vi "tdmsGenToolAllDataTypes.vi"() -> ()   [LabVIEW 2026]
uses:
  <vilib>/platform/TimedLoop/XDataNode/XDataNode.xnode
  <vilib>/Platform/TimedLoop/XDataNode/nitl_modes.ctl
  <vilib>/Platform/TimedLoop/XDataNode/XDNodeRunTimeDep.lvlib
  <vilib>/Platform/TimedLoop/XDataNode/wakeup.ctl
  <vilib>/Platform/TimedLoop/XDataNode/timing_clust.ctl
  <vilib>/DAQmx/configure/timing.llb/DAQmx Timing (Sample Clock).vi
  <vilib>/DAQmx/configure/task.llb/DAQmx Configure Logging (TDMS).vi
  <vilib>/DAQmx/create/channels.llb/DAQmx Create Channel (AI-Voltage-Basic).vi
panel:
  in  "physical channels 2":tag
  in  "number of loops":i32=1
  in  "file format version (2.0)":enum16{"1.0", "2.0"}(ring)=enum."2.0"
  in  "create index file? (T)":bool=TRUE
  in  "byte order (2:little-endian)":T1(ring)
  in  "physical channels":tag[](array[tag])
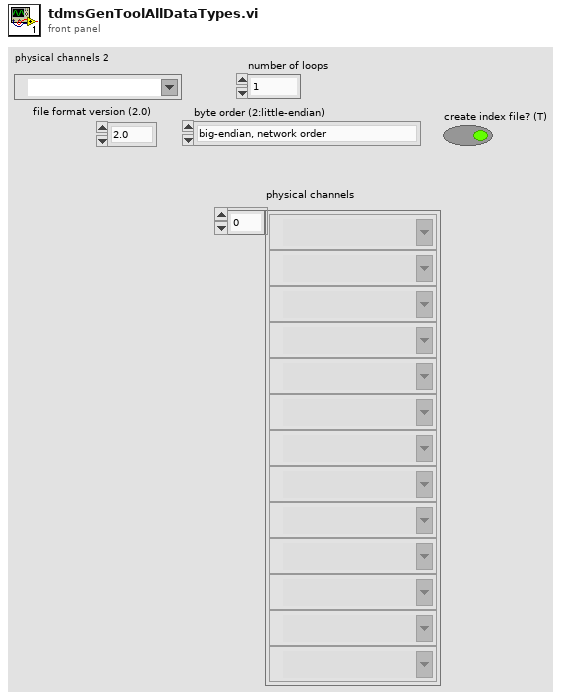
[diagram p1: front panel]
types:
  T1 = enum16{"big-endian, network order", "native, host order", "little-endian"}
  T2 = enum16{"open", "open or create", "create or replace", "create", "open (read-only)"}
  T3 = typedef "XDNodeRunTimeDep.lvlib/nitl_modes.ctl" = enum32{"No Change", "Process missed periods, maintain original phase", "Discard missed periods, maintain original phase", "Process missed periods, ignore original phase", "Discard missed periods, ignore original phase"}
  T4 = typedef "XDNodeRunTimeDep.lvlib/timing_clust.ctl" = cluster{"Expected End [f-1]":u64, "Actual End [f-1]":u64, "Finished Late? [f-1]":bool, "Expected End [i-1]":u64, "Actual End [i-1]":u64, "Finished Late? [i-1]":bool, "Expected Start [i]":u64, "Actual Start [i]":u64, "Expected Start [f]":u64, "Actual Start [f]":u64, "Source Name":string, "Structure Name":string, "Period":i64, "Deadline":i64, "Offset":i64, "Start":i64, "Priority":i32, "Timeout":i32, "Mode":T3, "Wakeup Reason":T5, "Error":errorcluster, "Source Type":string, "Secondary Source Type":string, "Global End Time":u64, "Global Start Time":u64, "Frame Duration":u64, "Iteration Duration":u64, "Assigned CPU":i32, "I/O Scan Engine Mode":u32}
  T5 = typedef "XDNodeRunTimeDep.lvlib/wakeup.ctl" = enum32{"Normal", "Aborted", "Asynchronous wakeup", "Timing source error", "Timed loop error", "Timeout"}
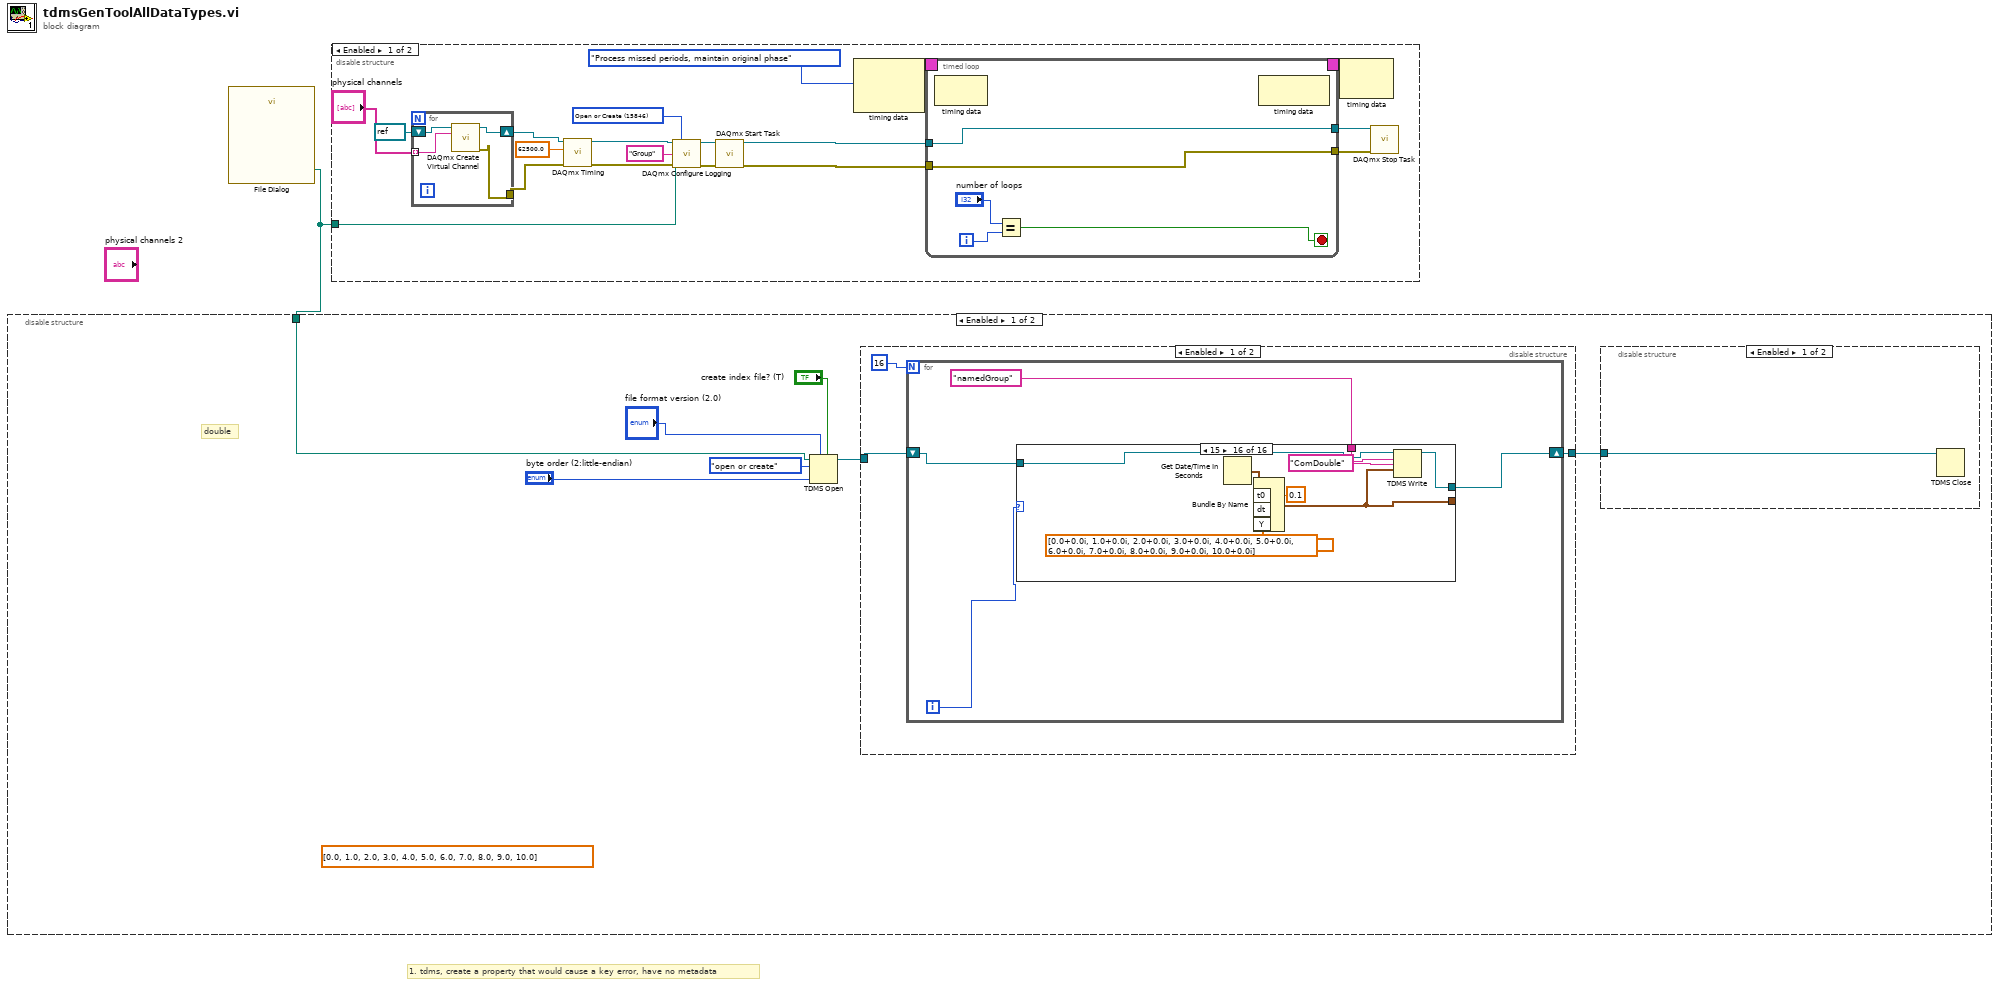
[diagram p0: block diagram]
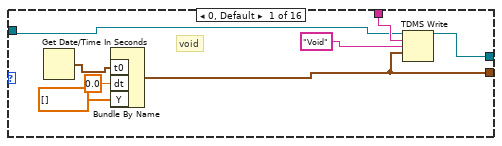
[diagram p3: hidden frame]
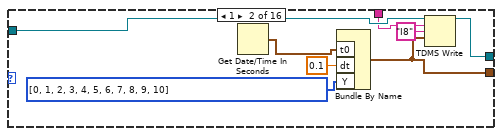
[diagram p4: hidden frame]
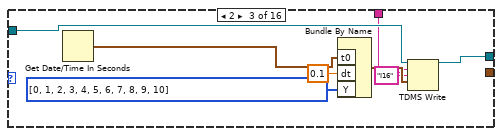
[diagram p5: hidden frame]
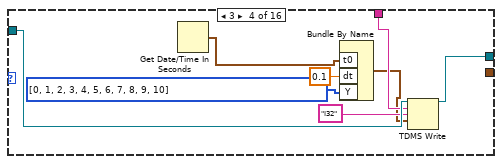
[diagram p6: hidden frame]
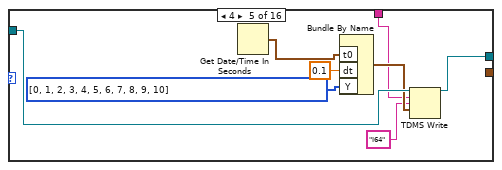
[diagram p7: hidden frame]
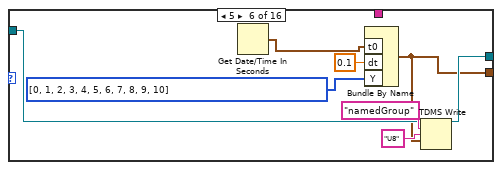
[diagram p8: hidden frame]
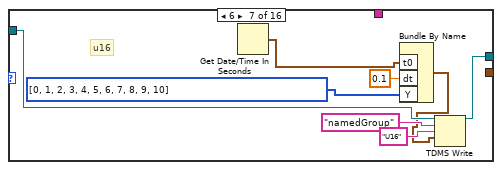
[diagram p9: hidden frame]
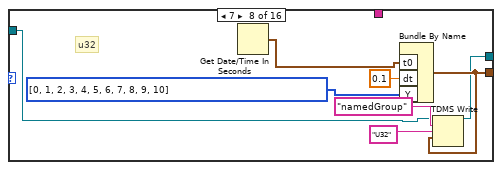
[diagram p10: hidden frame]
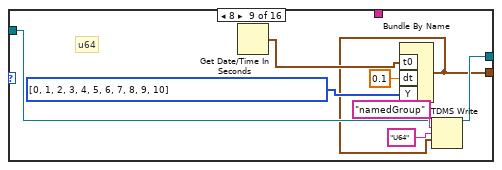
[diagram p11: hidden frame]
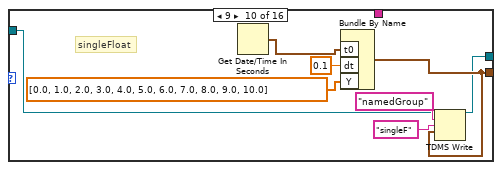
[diagram p12: hidden frame]
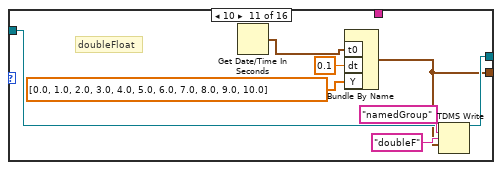
[diagram p13: hidden frame]
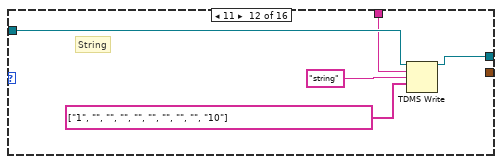
[diagram p14: hidden frame]
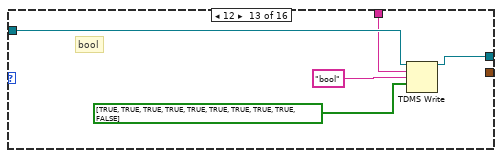
[diagram p15: hidden frame]
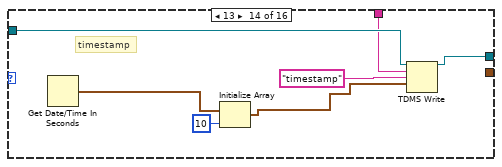
[diagram p16: hidden frame]
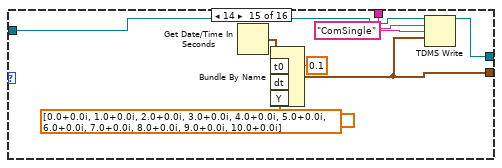
[diagram p17: hidden frame]
diagram:
  # "1. tdms, create a property that would cause a key error, have no metadata"
  n1 = call "File Dialog"() -> ("selected path"=w1:path)  [unwired: 12 in, 3 out]
  n2 = disable-structure shown="Enabled" {
    disable-tunnel: w1 -> [w6 _]
    frame Enabled {
      (unwired) sgl[] [0.0, 1.0, 2.0, 3.0, 4.0, 5.0, 6.0, 7.0, 8.0, 9.0, 10.0] ("Y")
      # "double"
      n3 = TDMS Open(5:"create index file? (T)", 7:"file format version (2.0)", 9:"byte order (2:little-endian)", 10:T2."open or create" ("operation (0:open)"), 11:w6) -> (3:w8:refnum<k34>)  [unwired: 2 in, 1 out]
      n4 = disable-structure shown="Enabled" {
        disable-tunnel: w8 -> [w11 w137]
        disable-tunnel: [w10 w137] -> w2
        frame Enabled {
          n5 = for {
            N: 16 -> [_]
            shift-right: [w14] -> w10
            shift-left: w11 -> [w15]
            i -> [w12]
            n6 = case shown="15" w12 {
              tunnel: [w19 w28 _ _ _ w56 _ w74 w80 w90 w96 _ _ _ w121 w129] -> _
              tunnel: w15 -> [w16 w26 w35 w44 w52 w58 w66 w72 w82 w88 w97 w107 w113 w120 w125 w133]
              tunnel: [w17 w27 w34 w43 w51 w57 w65 w73 w81 w89 w98 w106 w112 w119 w126 w134] -> w14
              tunnel: "namedGroup" ("group name in (Untitled)") -> [w20 w25 w33 w42 w49 _ _ _ _ _ _ w105 w111 w118 w124 w132]
              frame 0, Default {
                # "void"
                n7 = Get Date/Time In Seconds() -> (seconds since 1Jan1904=w23:timestamp)
                n8 = Bundle By Name("t0"=w23, "dt"=0.0, "Y"=dbl[] []) -> (w19:waveform(dbl))  [unwired: 1 in]
                n9 = TDMS Write(0:w16, 5:w20, 7:"Void", 9:w19) -> (4:w17:refnum<k34>)  [unwired: 2 in, 3 out]
              }
              frame 1 {
                n10 = Get Date/Time In Seconds() -> (seconds since 1Jan1904=w31:timestamp)
                n11 = Bundle By Name("t0"=w31, "dt"=0.1, "Y"=i8[] [0, 1, 2, 3, 4, 5, 6, 7, 8, 9, 10]) -> (w28:waveform(i8))  [unwired: 1 in]
                n12 = TDMS Write(0:w26, 5:w25, 7:"I8" ("channel name(s) in (Untitled)"), 9:w28) -> (4:w27:refnum<k34>)  [unwired: 2 in, 3 out]
              }
              frame 2 {
                n13 = Get Date/Time In Seconds() -> (seconds since 1Jan1904=w39:timestamp)
                n14 = Bundle By Name("t0"=w39, "dt"=0.1, "Y"=i16[] [0, 1, 2, 3, 4, 5, 6, 7, 8, 9, 10]) -> (w36:waveform(i16))  [unwired: 1 in]
                n15 = TDMS Write(0:w35, 5:w33, 7:"I16" ("channel name(s) in (Untitled)"), 9:w36) -> (4:w34:refnum<k34>)  [unwired: 2 in, 3 out]
              }
              frame 3 {
                n16 = Get Date/Time In Seconds() -> (seconds since 1Jan1904=w47:timestamp)
                n17 = Bundle By Name("t0"=w47, "dt"=0.1, "Y"=i32[] [0, 1, 2, 3, 4, 5, 6, 7, 8, 9, 10]) -> (w40:waveform(i32))  [unwired: 1 in]
                n18 = TDMS Write(0:w44, 5:w42, 7:"I32" ("group name in (Untitled)"), 9:w40) -> (4:w43:refnum<k34>)  [unwired: 2 in, 3 out]
              }
              frame 4 {
                n19 = Get Date/Time In Seconds() -> (seconds since 1Jan1904=w55:timestamp)
                n20 = Bundle By Name("t0"=w55, "dt"=0.1, "Y"=i64[] [0, 1, 2, 3, 4, 5, 6, 7, 8, 9, 10]) -> (w50:waveform(i64))  [unwired: 1 in]
                n21 = TDMS Write(0:w52, 5:w49, 7:"I64" ("group name in (Untitled)"), 9:w50) -> (4:w51:refnum<k34>)  [unwired: 2 in, 3 out]
              }
              frame 5 {
                n22 = Get Date/Time In Seconds() -> (seconds since 1Jan1904=w63:timestamp)
                n23 = Bundle By Name("t0"=w63, "dt"=0.1, "Y"=u8[] [0, 1, 2, 3, 4, 5, 6, 7, 8, 9, 10]) -> (w56:waveform(u8))  [unwired: 1 in]
                n24 = TDMS Write(0:w58, 5:"namedGroup" ("group name in (Untitled)"), 7:"U8" ("group name in (Untitled)"), 9:w56) -> (4:w57:refnum<k34>)  [unwired: 2 in, 3 out]
              }
              frame 6 {
                # "u16"
                n25 = Get Date/Time In Seconds() -> (seconds since 1Jan1904=w71:timestamp)
                n26 = Bundle By Name("t0"=w71, "dt"=0.1, "Y"=u16[] [0, 1, 2, 3, 4, 5, 6, 7, 8, 9, 10]) -> (w64:waveform(u16))  [unwired: 1 in]
                n27 = TDMS Write(0:w66, 5:"namedGroup" ("group name in (Untitled)"), 7:"U16" ("group name in (Untitled)"), 9:w64) -> (4:w65:refnum<k34>)  [unwired: 2 in, 3 out]
              }
              frame 7 {
                # "u32"
                n28 = Get Date/Time In Seconds() -> (seconds since 1Jan1904=w79:timestamp)
                n29 = Bundle By Name("t0"=w79, "dt"=0.1, "Y"=u32[] [0, 1, 2, 3, 4, 5, 6, 7, 8, 9, 10]) -> (w74:waveform(u32))  [unwired: 1 in]
                n30 = TDMS Write(0:w72, 5:"namedGroup" ("group name in (Untitled)"), 7:"U32" ("group name in (Untitled)"), 9:w74) -> (4:w73:refnum<k34>)  [unwired: 2 in, 3 out]
              }
              frame 8 {
                # "u64"
                n31 = Get Date/Time In Seconds() -> (seconds since 1Jan1904=w87:timestamp)
                n32 = Bundle By Name("t0"=w87, "dt"=0.1, "Y"=u64[] [0, 1, 2, 3, 4, 5, 6, 7, 8, 9, 10]) -> (w80:waveform(u64))  [unwired: 1 in]
                n33 = TDMS Write(0:w82, 5:"namedGroup" ("group name in (Untitled)"), 7:"U64" ("group name in (Untitled)"), 9:w80) -> (4:w81:refnum<k34>)  [unwired: 2 in, 3 out]
              }
              frame 9 {
                # "singleFloat"
                n34 = Get Date/Time In Seconds() -> (seconds since 1Jan1904=w95:timestamp)
                n35 = Bundle By Name("t0"=w95, "dt"=0.1, "Y"=sgl[] [0.0, 1.0, 2.0, 3.0, 4.0, 5.0, 6.0, 7.0, 8.0, 9.0, 10.0]) -> (w90:waveform(sgl))  [unwired: 1 in]
                n36 = TDMS Write(0:w88, 5:"namedGroup" ("group name in (Untitled)"), 7:"singleF" ("group name in (Untitled)"), 9:w90) -> (4:w89:refnum<k34>)  [unwired: 2 in, 3 out]
              }
              frame 10 {
                # "doubleFloat"
                n37 = Get Date/Time In Seconds() -> (seconds since 1Jan1904=w103:timestamp)
                n38 = Bundle By Name("t0"=w103, "dt"=0.1, "Y"=dbl[] [0.0, 1.0, 2.0, 3.0, 4.0, 5.0, 6.0, 7.0, 8.0, 9.0, 10.0]) -> (w96:waveform(dbl))  [unwired: 1 in]
                n39 = TDMS Write(0:w97, 5:"namedGroup" ("group name in (Untitled)"), 7:"doubleF" ("group name in (Untitled)"), 9:w96) -> (4:w98:refnum<k34>)  [unwired: 2 in, 3 out]
              }
              frame 11 {
                # "String"
                n40 = TDMS Write(0:w107, 5:w105, 7:"string" ("channel name(s) in (Untitled)"), 9:string[] ["1", "", "", "", "", "", "", "", "", "10"] ("Y")) -> (4:w106:refnum<k34>)  [unwired: 2 in, 3 out]
              }
              frame 12 {
                # "bool"
                n41 = TDMS Write(0:w113, 5:w111, 7:"bool" ("channel name(s) in (Untitled)"), 9:bool[] [TRUE, TRUE, TRUE, TRUE, TRUE, TRUE, TRUE, TRUE, TRUE, FALSE]) -> (4:w112:refnum<k34>)  [unwired: 2 in, 3 out]
              }
              frame 13 {
                # "timestamp"
                n42 = Get Date/Time In Seconds() -> (seconds since 1Jan1904=w116:timestamp)
                n43 = Initialize Array(w116, 10 ("dimension size")) -> (w114:timestamp[])
                n44 = TDMS Write(0:w120, 5:w118, 7:"timestamp" ("channel name(s) in (Untitled)"), 9:w114) -> (4:w119:refnum<k34>)  [unwired: 2 in, 3 out]
              }
              frame 14 {
                n45 = Get Date/Time In Seconds() -> (seconds since 1Jan1904=w128:timestamp)
                n46 = Bundle By Name("t0"=w128, "dt"=0.1, "Y"=csg[] [0.0+0.0i, 1.0+0.0i, 2.0+0.0i, 3.0+0.0i, 4.0+0.0i, 5.0+0.0i, 6.0+0.0i, 7.0+0.0i, 8.0+0.0i, 9.0+0.0i, 10.0+0.0i]) -> (w121:waveform(csg))  [unwired: 1 in]
                n47 = TDMS Write(0:w125, 5:w124, 7:"ComSingle" ("channel name(s) in (Untitled)"), 9:w121) -> (4:w126:refnum<k34>)  [unwired: 2 in, 3 out]
              }
              frame 15 {
                n48 = Get Date/Time In Seconds() -> (seconds since 1Jan1904=w136:timestamp)
                n49 = Bundle By Name("t0"=w136, "dt"=0.1, "Y"=cdb[] [0.0+0.0i, 1.0+0.0i, 2.0+0.0i, 3.0+0.0i, 4.0+0.0i, 5.0+0.0i, 6.0+0.0i, 7.0+0.0i, 8.0+0.0i, 9.0+0.0i, 10.0+0.0i]) -> (w129:waveform(cdb))  [unwired: 1 in]
                n50 = TDMS Write(0:w133, 5:w132, 7:"ComDouble" ("channel name(s) in (Untitled)"), 9:w129) -> (4:w134:refnum<k34>)  [unwired: 2 in, 3 out]
              }
            }
          }
        }
        frame Disabled {
        }
      }
      n51 = disable-structure shown="Enabled" {
        disable-tunnel: w2 -> [w138 _]
        frame Enabled {
          n52 = TDMS Close(11:w138) -> ()  [unwired: 1 in, 2 out]
        }
        frame Disabled {
        }
      }
    }
    frame Disabled {
    }
  }
  n53 = disable-structure shown="Enabled" {
    disable-tunnel: w1 -> [w143 _]
    frame Enabled {
      w154 = 15846 items=["Open"=10437, "Open or Create"=15846, "Create or Replace"=15847, "Create"=15848] ("operation")
      n54 = for {
        tunnel: [w160] -> w141
        tunnel: "physical channels" -> [w159] mode=indexing
        shift-right: [w161] -> w142
        shift-left: refnum<k21> refnum ("task out") -> [w158]
        n55 = call-poly <vilib>:"DAQmx Create Virtual Channel.vi"("task in"=w158, "physical channels"=w159) -> ("task out"=w161:refnum<k21>, "error out"=w160:errorcluster)  [unwired: 12 in]
      }
      n56 = call-poly <vilib>:"DAQmx Timing.vi"("task/channels in"=w142, "rate"=62500.0, "error in"=w141) -> ("task out"=w152:refnum<k21>, "error out"=w151:errorcluster)  [unwired: 11 in]
      n57 = call-poly <vilib>:"DAQmx Configure Logging.vi"("task/channels in"=w152, "operation"=w154, "file path"=w143, "group name"="Group", "error in"=w151) -> ("task out"=w150:refnum<k21>, "error out"=w149:errorcluster)  [unwired: 9 in]
      n58 = call <vilib>:"DAQmx Start Task.vi"("task/channels in"=w150, "error in"=w149) -> ("task out"=w148:refnum<k21>, "error out"=w147:errorcluster)  [unwired: 12 in]
      n59 = node-c288(nitl_modes."Process missed periods, maintain original phase" ("Mode")) -> (w157:T4)  [unwired: 1 in]
      n60 = timed-loop {
        tunnel: w148 -> [w164]
        tunnel: w147 -> [w163]
        timing: w157 -> [_]
        timing-out: [_] -> w156
        tunnel: [w164] -> w146
        tunnel: [w163] -> w145
        i -> [w166]
        stop <- w165 stop-if-true
        n61 = node-c288() -> ()  [unwired: 1 in, 1 out]
        n62 = Equal?(x="number of loops", y=w166) -> (x = y?=w165:bool)
        n63 = node-c288() -> ()  [unwired: 1 in, 1 out]
      }
      n64 = node-c288(w156) -> ()  [unwired: 1 out]
      n65 = call <vilib>:"DAQmx Stop Task.vi"("task/channels in"=w146, "error in"=w145) -> ()  [unwired: 12 in, 2 out]
    }
    frame Disabled {
    }
  }
